vi "DHE_SetGeometry.vi"(0 "refnum":i32=2048, 5 "modifiers":string, 11 "error in (no error)":errorcluster) -> (4 "fd out":i32, 6 "return value":i32, 8 "X total size":u16, 10 "Y total size":u16, 14 "DET_READ_TIME":sgl=3.5 format="%.2f", 15 "error out":errorcluster)   [LabVIEW 2016]
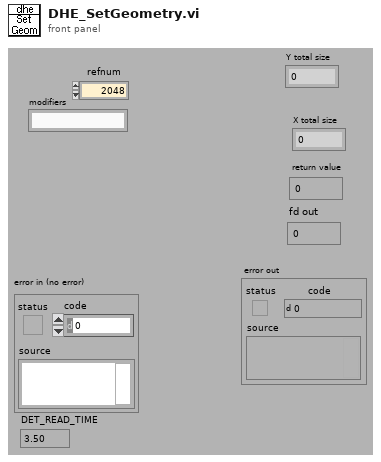
[diagram p1: front panel]
types:
  T1 = typedef "GEOM_CorrectedFPA.ctl" = cluster{"readmode":string, "amplifiers":cluster{"number":i32, "xstart":i32, "ystart":i32}[], "totxsize":i32, "totysize":i32, "maxxdim":i32, "maxydim":i32, "numxamps":i32, "numyamps":i32, "totxdata":i32, "totydata":i32, "xdataamp":i32, "ydataamp":i32, "totpixels":i32}
  T2 = typedef "GEOM_Amplifier.ctl" = cluster{"number":i32, "type":T3, "rotated":i16, "fliped":u16, "FPAcoord":cluster{"xstart":i32, "ystart":i32}, "Physical_size":cluster{"columns":i32, "rows":i32}, "predata":cluster{"columns":i32, "rows":i32}, "postdata":cluster{"columns":i32, "rows":i32}, "Req ROIs":T4, "Corr ROI":T4, "Detnumber":i32, "ampID":string, "discard":i32}
  T3 = typedef "GEOM_AmpType.ctl" = u16
  T4 = typedef "GEOM_ROI.ctl" = T5[]
  T5 = typedef "GEOM_Coords.ctl" = cluster{"xstart":u32, "ystart":u32, "xsize":u32, "ysize":u32}
  T6 = typedef "DatabaseHand_RefNum.ctl" = refnum<vi>
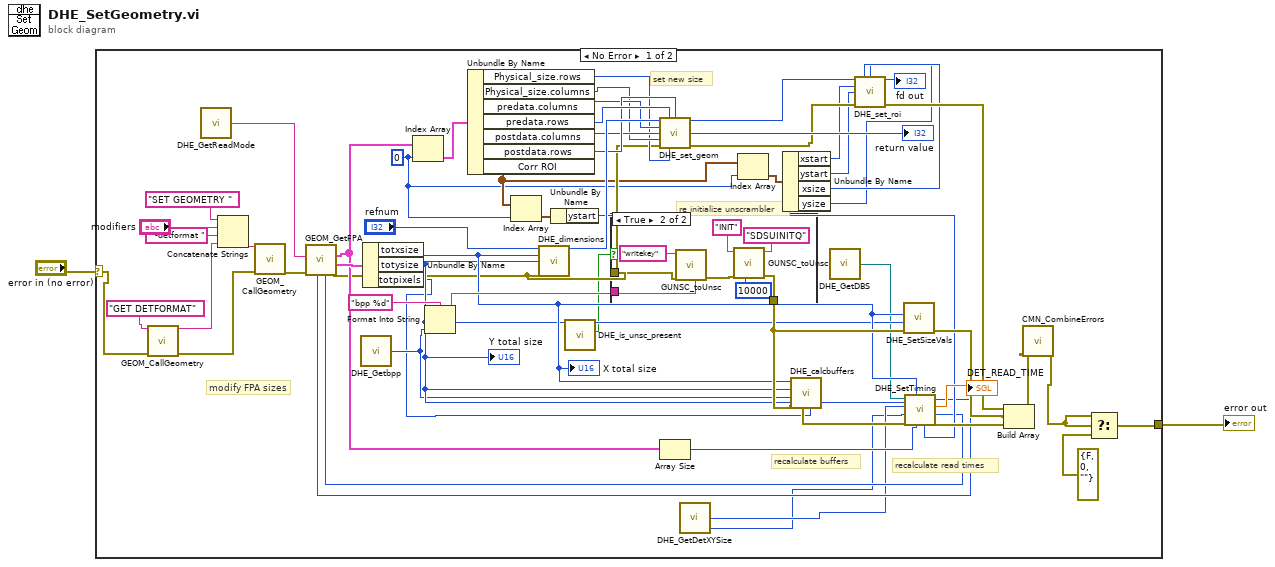
[diagram p0: block diagram]
diagram:
  n1 = case shown="No Error" "error in (no error)" {
    selector: "error in (no error)" -> [w15 w70]
    tunnel: [w32 w70] -> w1
    frame No Error {
      w9 = 0 ("index")
      # "recalculate read times"
      # "recalculate buffers"
      # "re initialize unscrambler"
      # "set new size"
      # "modify FPA sizes"
      n2 = call "GEOM_CallGeometry.vi"("Command"="GET DETFORMAT", "error in (no error)"=w15) -> ("ImmedReplyString"=w16:string, "error out"=w14:errorcluster)  [unwired: 12 out]
      n3 = call "DHE_GetReadMode.vi"() -> ("DHE_ReadMode"=w25:string)  [unwired: 9 out]
      n4 = Concatenate Strings("SET GEOMETRY " ("Command"), "modifiers", " -detformat " ("string"), w16) -> (w59:string)
      n5 = call "GEOM_CallGeometry.vi"("Command"=w59, "error in (no error)"=w14) -> ("error out"=w58:errorcluster)  [unwired: 13 out]
      n6 = call "GEOM_GetFPA.vi"("error in (no error)"=w58, "readmode"=w25) -> ("error out"=w21:errorcluster, "CorrectedFPACoord"=w56:T1, "amplifiers"=w45:T2[], "numyamps"=w27:i32, "numxamps"=w28:i32)  [unwired: 1 in, 4 out]
      n7 = call "DHE_Getbpp.vi"() -> ("DHE_bpp"=w24:i32)  [unwired: 9 out]
      n8 = Unbundle By Name(w56) -> ("totxsize"=w48:i32, "totysize"=w47:i32, "totpixels"=w19:i32)
      "Y total size" <- w47
      "X total size" <- w48
      n9 = Index Array(array=w45, index=w9) -> (element=w44:T2)
      n10 = Format Into String(format string="bpp %d", w24) -> (resulting string=w50:string)  [unwired: 2 in, 1 out]
      n11 = Unbundle By Name(w44) -> ("Physical_size.rows"=w38:i32, "Physical_size.columns"=w39:i32, "predata.columns"=w41:i32, "predata.rows"=w43:i32, "postdata.columns"=w40:i32, "postdata.rows"=w42:i32, "Corr ROI"=w10:T4)
      n12 = Index Array(array=w10, index=w9) -> (element=w31:T5)
      n13 = call "DHE_dimensions.vi"("fd"="refnum", "Columns"=w48, "Rows"=w47, "error in (no error)"=w21) -> ("fd out"=w46:i32)  [unwired: 11 out]
      n14 = Unbundle By Name(w31) -> ("ystart"=w29:u32)
      n15 = call "DHE_is_unsc_present.vi"() -> ("value"=w20:bool)  [unwired: 1 in, 10 out]
      n16 = case shown="True" w20 {
        tunnel: [w61 w66] -> w51
        tunnel: w50 -> [_ w63]
        tunnel: w21 -> [w61 w62]
        frame False {
        }
        frame True {
          n17 = call "GUNSC_toUnsc.vi"("key"=w63, "error in (no error)"=w62, "command"="writekey") -> ("error out"=w65:errorcluster)  [unwired: 6 in, 2 out]
          n18 = call "GUNSC_toUnsc.vi"("responseQ"="SDSUINITQ", "bpp"=10000 ("ms timeout (-1)"), "error in (no error)"=w65, "command"="INIT") -> ("error out"=w66:errorcluster)  [unwired: 5 in, 2 out]
        }
      }
      n19 = call "DHE_set_geom.vi"("fd"=w46, "ypredata"=w43, "ypostdata"=w42, "xpredata"=w41, "xpostdata"=w40, "xdata"=w39, "error in (no error)"=w21, "ydata"=w38) -> ("fd out"=w12:i32, "return value"=→"return value":i32, "error out"=w13:errorcluster)  [unwired: 5 out]
      n20 = Array Size(array=w45) -> (size(s)=w49:i32)
      n21 = call "DHE_GetDetXYSize.vi"() -> ("DHE_DetYsize"=w23:i32, "DHE_DetXsize"=w22:i32)  [unwired: 8 out]
      n22 = Index Array(array=w10, index=w9) -> (element=w8:T5)
      n23 = Unbundle By Name(w8) -> ("xstart"=w6:u32, "ystart"=w5:u32, "xsize"=w4:u32, "ysize"=w3:u32)
      n24 = call "DHE_calcbuffers.vi"("totpixelsin"=w19, "error in (no error)"=w51, "bpp"=w24, "nrows"=w47, "ncols"=w48) -> ("error out"=w53:errorcluster)  [unwired: 1 in, 5 out]
      n25 = call "DHE_GetDBS.vi"() -> ("DHE_DBSRef"=w26:T6)  [unwired: 9 out]
      n26 = call "DHE_set_roi.vi"("fd"=w12, "xlenght"=w4, "ylenght"=w3, "xstart"=w6, "ystart"=w5, "error in (no error)"=w13) -> ("fd out"=→"fd out":i32, "error out"=w7:errorcluster)  [unwired: 8 out]
      n27 = call "DHE_SetSizeVals.vi"("error in"=w51, "ytotsize"=w47, "xtotsize"=w48) -> ("errorout"=w36:errorcluster)  [unwired: 8 out]
      n28 = call "DHE_SetTiming.vi"("num of Y amps"=w27, "num of X amps"=w28, "yroi start"=w29, "roi rows"=w47, "Num of amps"=w49, "roi cols"=w48, "error in"=w53, "totysize"=w22, "totxsize"=w23, "Database RefNum out"=w26) -> ("errorout"=w37:errorcluster, "DET_READ_TIME"=→"DET_READ_TIME":sgl)
      n29 = Build Array(w7, w36, w37) -> (w35:errorcluster[])
      n30 = call "CMN_CombineErrors.vi"("Errors"=w35) -> ("error out"=w33:errorcluster)  [unwired: 10 out]
      n31 = Select(t=w33, s=w33, f=errorcluster {"status"=FALSE, "code"=0, "source"=""}) -> (s? t:f=w32:errorcluster)
    }
    frame Error {
    }
  }
  "error out" <- w1
